vi "Set Selection Font by Name Size and Style.vi"(7 "newStyle":i32(ring) items=["Regular"=0, "Bold"=1, "Italic"=2, "Underline"=4, "Strikeout"=8], 8 "error in (no error)":errorcluster caption="错误输入（无错误）", 9 "emSize":sgl, 10 "familyName":string, 11 "RichText 输入":refnum<class "RichText.lvclass"> caption="DNL_LabVIEW Object in") -> (0 "error out":errorcluster caption="错误输出", 3 "RichText 输出":refnum<class "RichText.lvclass"> caption="DNL_LabVIEW Object out")   [LabVIEW 2012, in "RichText.lvclass"]
uses:
  RichText.lvclass
  RichText.lvclass/RichText.ctl
  System.Drawing
  System.Windows.Forms
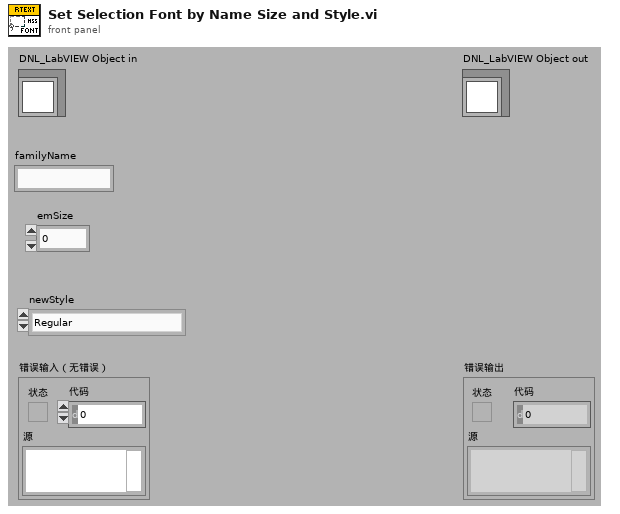
[diagram p1: front panel]
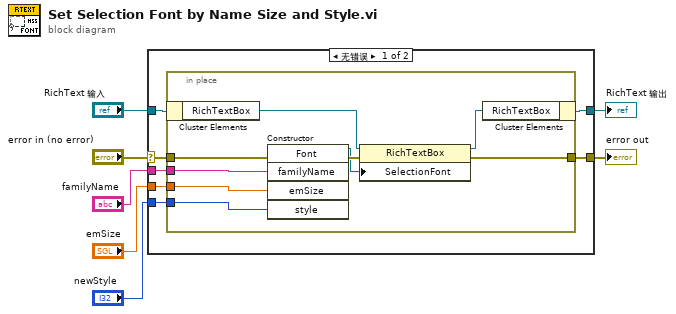
[diagram p0: block diagram]
diagram:
  n1 = case shown="无错误" "error in (no error)" {
    selector: "error in (no error)" -> [w11 w25]
    tunnel: [w10 w25] -> w6
    tunnel: [w13 w24] -> w4
    tunnel: "RichText 输入" -> [w14 w24]
    tunnel: "newStyle" -> [w12 _]
    tunnel: "familyName" -> [w9 _]
    tunnel: "emSize" -> [w8 _]
    frame No Error {
      n2 = in-place {
        in-place-border: w12 -> [w19]
        in-place-border: w11 -> [w15]
        in-place-border: [w21] -> w10
        in-place-border: w9 -> [w18]
        in-place-border: w8 -> [w17]
        n3 = in-place-cluster #1(w14) -> ("RichTextBox"=w16:refnum<k24>)
        n4 = constructor class="Font"(error in=w15, "familyName"=w18, "emSize"=w17, "style"=w19) -> (reference out=w20:refnum<k24>, error out=w22:errorcluster)  [unwired: 2 in, 4 out]
        n5 = property class="RichTextBox"(reference=w16, error in=w22, "SelectionFont"=w20) -> (reference out=w23:refnum<k24>, error out=w21:errorcluster)
        n6 = in-place-cluster #1("RichTextBox"=w23) -> (w13:refnum<class "RichText.lvclass">)
      }
    }
    frame Error {
    }
  }
  "error out" <- w6
  "RichText 输出" <- w4
